vi "Wavelet.vi"(3 "Shifts, b":dbl[](array[numeric]) format="%.3f", 4 "Scales, a":dbl[](array[numeric]) format="%.3f", 5 "Instant, kT":dbl=1.0 min=1.0 max=10.0 step=1.0 format="%.3f", 6 "Activation function, fn":u16(ring) items=["Morlet", "RASP1", "RASP2", "RASP3", "POLYWOG1", "POLYWOG2", "POLYWOG3", "POLYWOG4", "POLYWOG5", "Shannon", "Atomic", "Flat top 1", "Flat top 2", "Flat top 3", "Flat top 4", "Flat top 5", "Flat top 6", "Hanning", "Hamming", "Blackman", "Blackman-Harris"]) -> (0 "Function, dy":dbl[](array[numeric]) format="%.3f", 1 "Function, y":dbl[](array[numeric]) format="%.3f", 2 "Tau, t":dbl[](array[numeric]) format="%.3f")   [LabVIEW 2022 SP3]
uses:
  <vilib>/express/express arith-compare/Formula/XNode/ExpressFormulaBlockNode.xnode
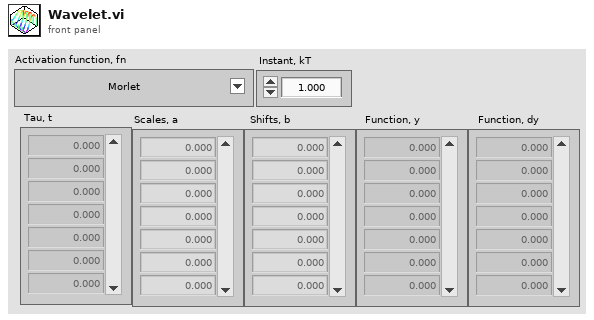
[diagram p1: front panel]
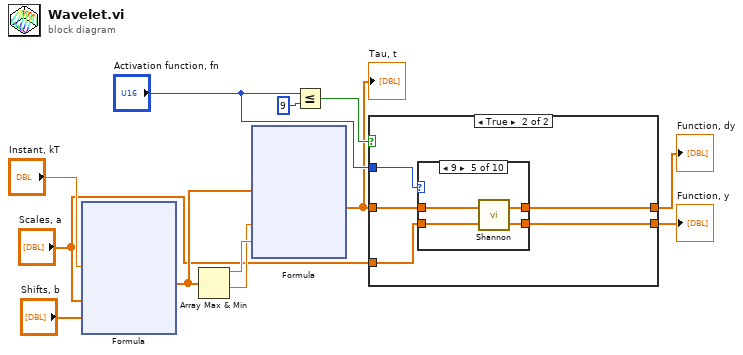
[diagram p0: block diagram]
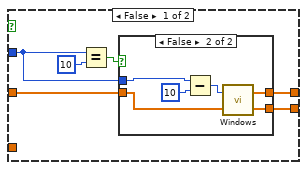
[diagram p2: hidden frame]
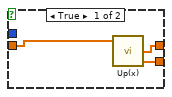
[diagram p3: hidden frame]
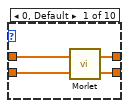
[diagram p4: hidden frame]
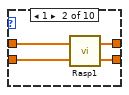
[diagram p5: hidden frame]
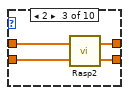
[diagram p6: hidden frame]
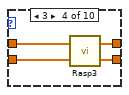
[diagram p7: hidden frame]
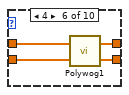
[diagram p8: hidden frame]
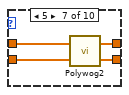
[diagram p9: hidden frame]
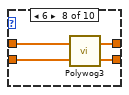
[diagram p10: hidden frame]
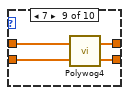
[diagram p11: hidden frame]
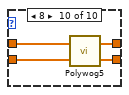
[diagram p12: hidden frame]
diagram:
  n1 = xnode "Formula"("instant"="Instant, kT", "scales"="Scales, a", "shifts"="Shifts, b") -> ("Result"=w7:dbl[])  [unwired: 1 in, 1 out]
  n2 = Array Max & Min(array=w7) -> (max value=w6:dbl, min value=w5:dbl)  [unwired: 2 out]
  n3 = xnode "Formula"("x"=w7, "min"=w5, "max"=w6) -> ("Result"=w2:dbl[])  [unwired: 1 in, 1 out]
  "Tau, t" <- w2
  n4 = Less Or Equal?(x="Activation function, fn", y=u16 9) -> (x <= y?=w11:bool)
  n5 = case shown="True" w11 {
    tunnel: "Activation function, fn" -> [w13 w32]
    tunnel: w2 -> [w16 w31]
    tunnel: "Scales, a" -> [_ w30]
    tunnel: [w15 w29] -> w9
    tunnel: [w14 w28] -> w8
    frame False {
      n6 = Equal?(x=w13, y=u16 10) -> (x = y?=w17:bool)
      n7 = case shown="False" w17 {
        tunnel: w16 -> [w21 w25]
        tunnel: [w20 w27] -> w15
        tunnel: [w19 w26] -> w14
        tunnel: w13 -> [_ w24]
        frame True {
          n8 = call "Up(x).vi"("Tau"=w21) -> ("dPsi"=w19:dbl[], "Psi"=w20:dbl[])
        }
        frame False {
          n9 = Subtract(x=w24, y=u16 10) -> (x-y=w22:u16)
          n10 = call "Windows.vi"("Tau"=w25, "WINDOW"=w22) -> ("dPsi"=w26:dbl[], "Psi"=w27:dbl[])
        }
      }
    }
    frame True {
      n11 = case shown="9" w32 {
        tunnel: w31 -> [w36 w40 w44 w48 w52 w55 w59 w64 w68 w72]
        tunnel: w30 -> [w35 w39 w43 w47 w51 w53 w60 w63 w67 w71]
        tunnel: [w34 w37 w42 w46 w50 w54 w58 w62 w66 w70] -> w29
        tunnel: [w33 w38 w41 w45 w49 w56 w57 w61 w65 w69] -> w28
        frame 0, Default {
          n12 = call "Morlet.vi"("z"=w35, "T"=w36) -> ("dY"=w33:dbl[], "Y"=w34:dbl[])
        }
        frame 1 {
          n13 = call "Rasp1.vi"("z"=w39, "T"=w40) -> ("dY"=w38:dbl[], "Y"=w37:dbl[])
        }
        frame 2 {
          n14 = call "Rasp2.vi"("z"=w43, "T"=w44) -> ("dY"=w41:dbl[], "Y"=w42:dbl[])
        }
        frame 3 {
          n15 = call "Rasp3.vi"("z"=w47, "T"=w48) -> ("dY"=w45:dbl[], "Y"=w46:dbl[])
        }
        frame 9 {
          n16 = call "Shannon.vi"("z"=w51, "T"=w52) -> ("dY"=w49:dbl[], "Y"=w50:dbl[])
        }
        frame 4 {
          n17 = call "Polywog1.vi"("z"=w53, "T"=w55) -> ("dY"=w56:dbl[], "Y"=w54:dbl[])
        }
        frame 5 {
          n18 = call "Polywog2.vi"("z"=w60, "T"=w59) -> ("dY"=w57:dbl[], "Y"=w58:dbl[])
        }
        frame 6 {
          n19 = call "Polywog3.vi"("z"=w63, "T"=w64) -> ("dY"=w61:dbl[], "Y"=w62:dbl[])
        }
        frame 7 {
          n20 = call "Polywog4.vi"("z"=w67, "T"=w68) -> ("dY"=w65:dbl[], "Y"=w66:dbl[])
        }
        frame 8 {
          n21 = call "Polywog5.vi"("z"=w71, "T"=w72) -> ("dY"=w69:dbl[], "Y"=w70:dbl[])
        }
      }
    }
  }
  "Function, y" <- w8
  "Function, dy" <- w9
